vi "Configure Generator Mode.vi"(8 "error in (no error)":errorcluster, 9 "Mode (CW)":i32(ring) items=["CW", "Dual Tone", "ARB"], 10 "Instance (1)":i32=1 format="%.0g", 11 "VISA resource name":refnum<visa-resource-name>) -> (0 "error out":errorcluster, 3 "VISA resource name out":refnum<visa-resource-name>)   [LabVIEW 2015, in "Rohde&Schwarz CMXP GPRF.lvlib"]
doc: "Selects generator mode.\n\nAttribute:\nRSCMXPGPRF_ATTR_BASEBAND_MODE\n\nRemote-control command:\nSOURce:GPRF:GEN<i>:BBMode"
uses:
  <instrlib>/Rohde&Schwarz CMXP GPRF/Rohde&Schwarz CMXP GPRF.lvlib
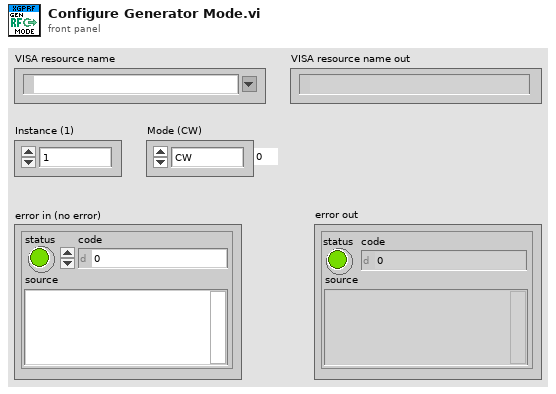
[diagram p1: front panel]
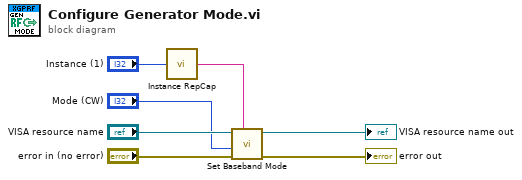
[diagram p0: block diagram]
diagram:
  n1 = call <instrlib>:"Instance RepCap.vi"("instance  in"="Instance (1)") -> ("instance out"=w7:string)
  n2 = call "Set Baseband Mode"("Repeated Capabilities"=w7, "error in (no error)"="error in (no error)", "Baseband Mode (0 - CW)"="Mode (CW)", "instrument handle"="VISA resource name") -> ("error out"=→"error out":errorcluster, "instrument handle out"=→"VISA resource name out":refnum<visa-resource-name>)  [unwired: 6 in]
